vi "Update display.vi"(0 "This VI":refnum<vi>, 5 "Display":refnum<vi>, 9 "input":string, 11 "error in":errorcluster) -> (4 "Display out":string[][](array[string]), 6 "Location Cluster out":T1, 8 "Display array":string[][](array[string]), 10 "Display string":string, 15 "Error Out":errorcluster)   [LabVIEW 2018]
uses:
  location cluster.ctl
  CAEN globals.vi
panel:
  out "selected string":string
  out "Selection Position":cluster{i32, i32}
  out "Last cursor pos":cluster{i32, i32}
  out "Highlighted lines":i32[](array[numeric])
  out "Highlighted text":string[](array[string])
  out "sections":T2(array[cluster])
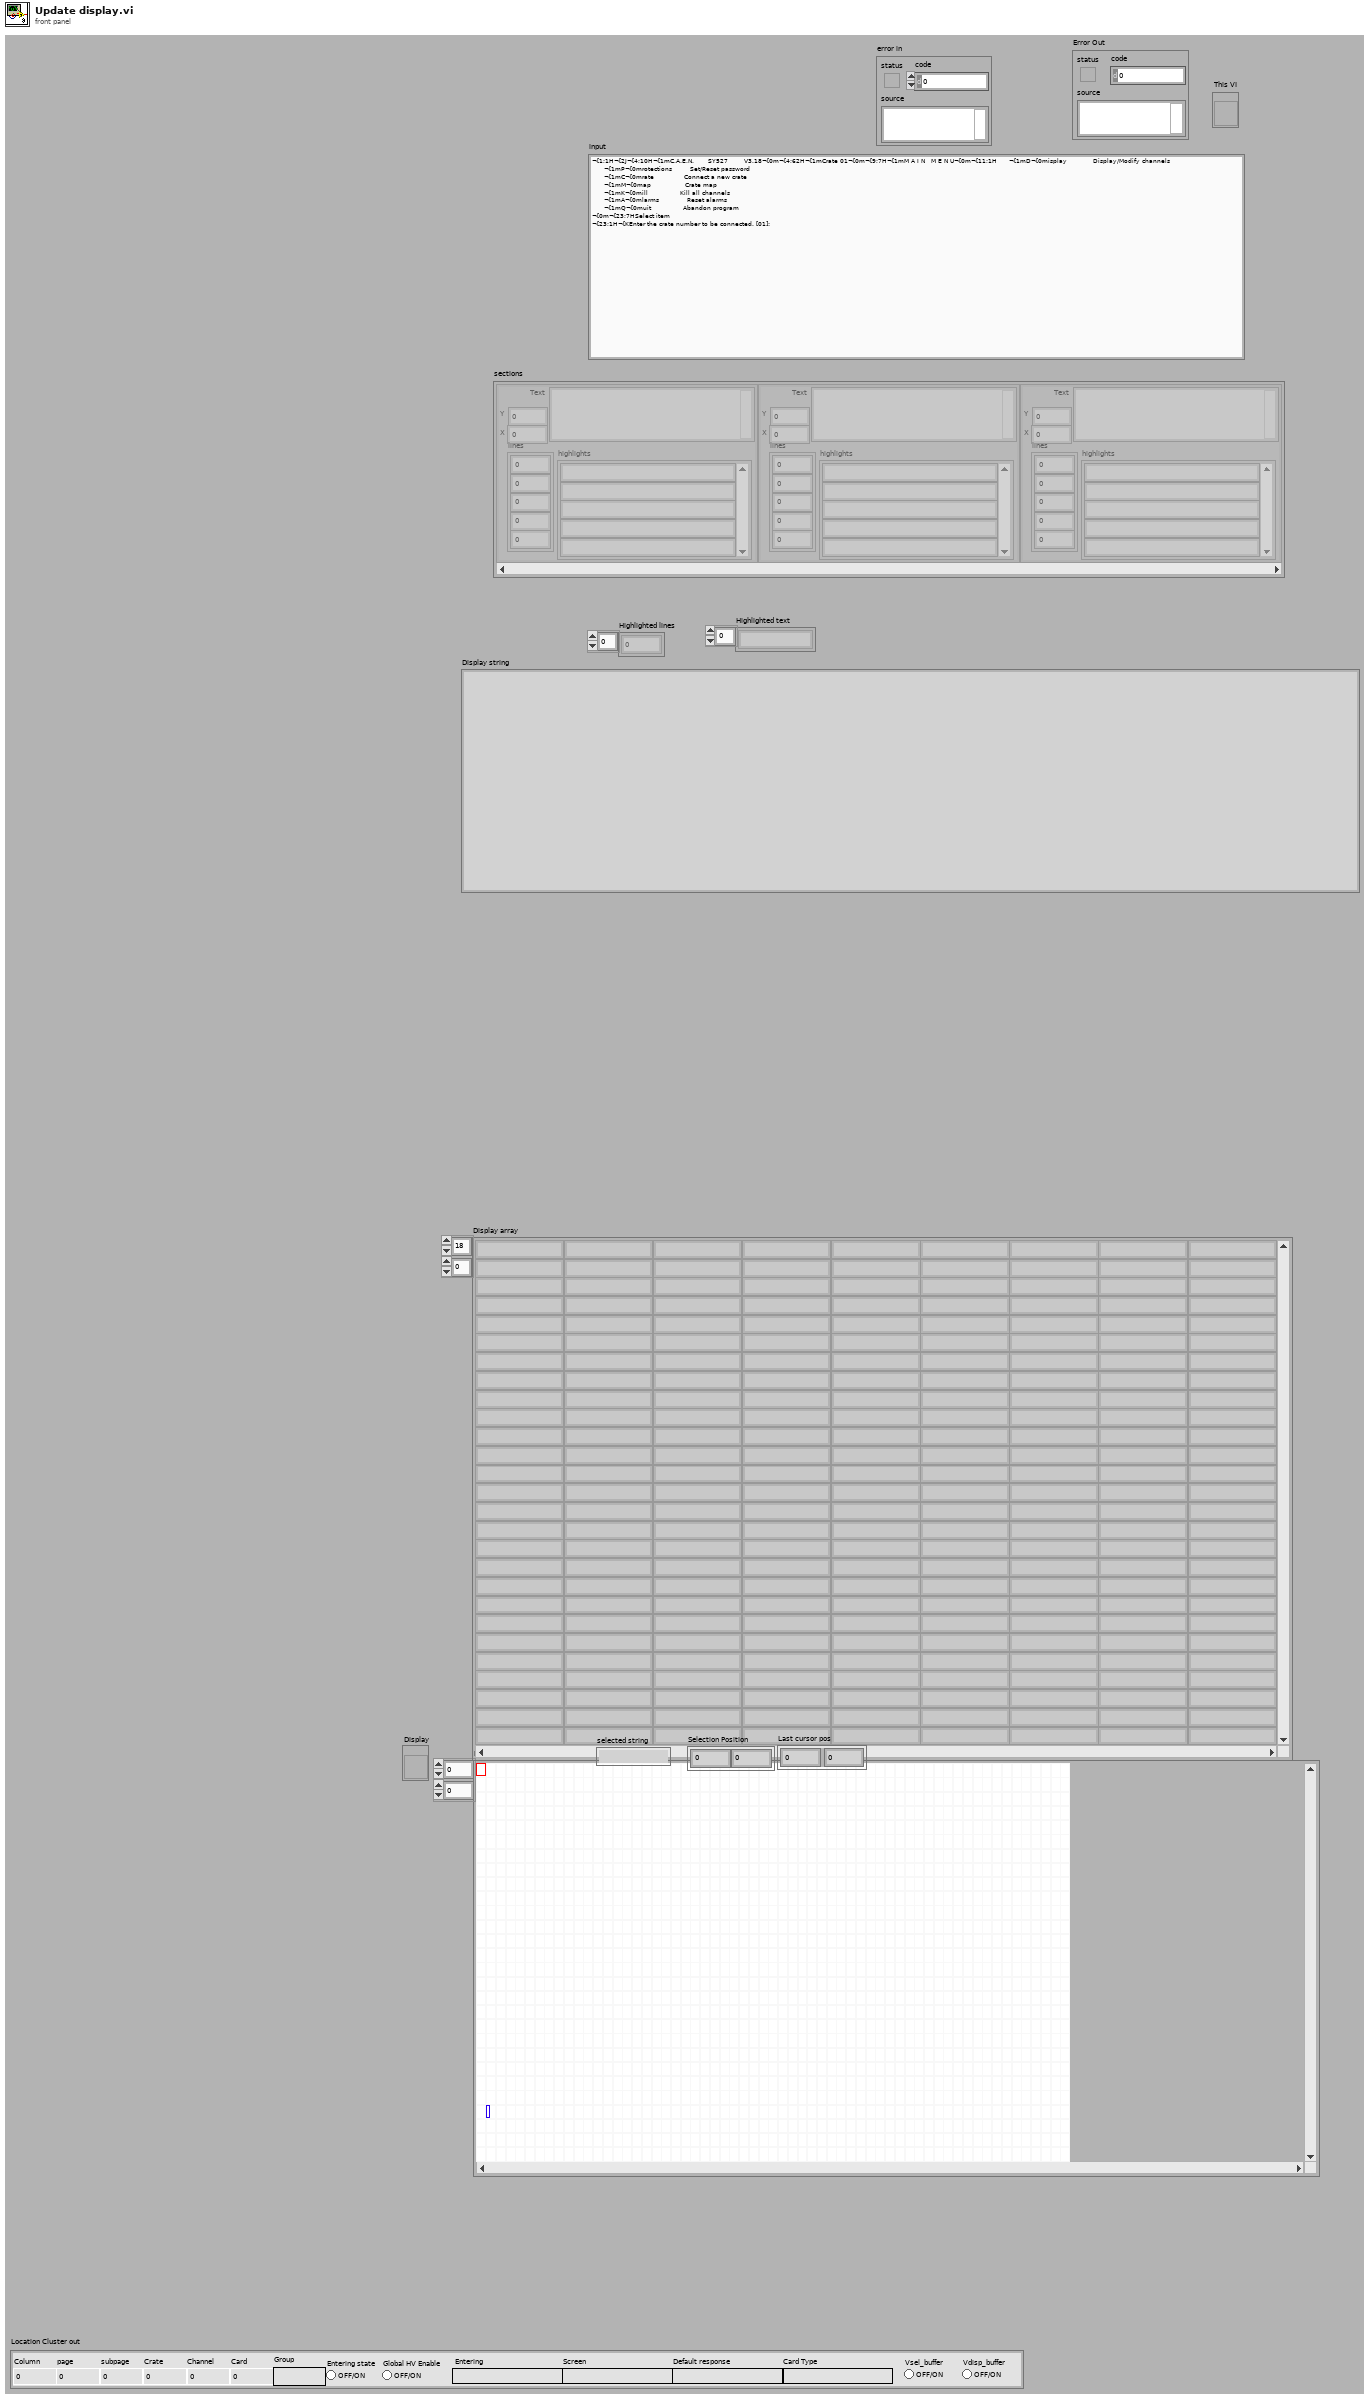
[diagram p1: front panel]
types:
  T1 = typedef "location cluster.ctl" = cluster{"Column":i32, "Card Type":string, "Channel":i32, "Card":i32, "Default response":string, "Entering":string, "Entering state":bool, "subpage":i32, "page":i32, "Crate":i32, "Screen":string, "Group":string, "Global HV Enable":bool, "Vsel_buffer":bool, "Vdisp_buffer":bool}
  T2 = cluster{"Y":i32, "X":i32, "Text":string, "highlights":string[], "lines":i32[]}[]
  T3 = cluster{"Y":i32, "X":i32, "stripped output":string, "highlighted strings":string[], "highlighted lines":i32[]}[]
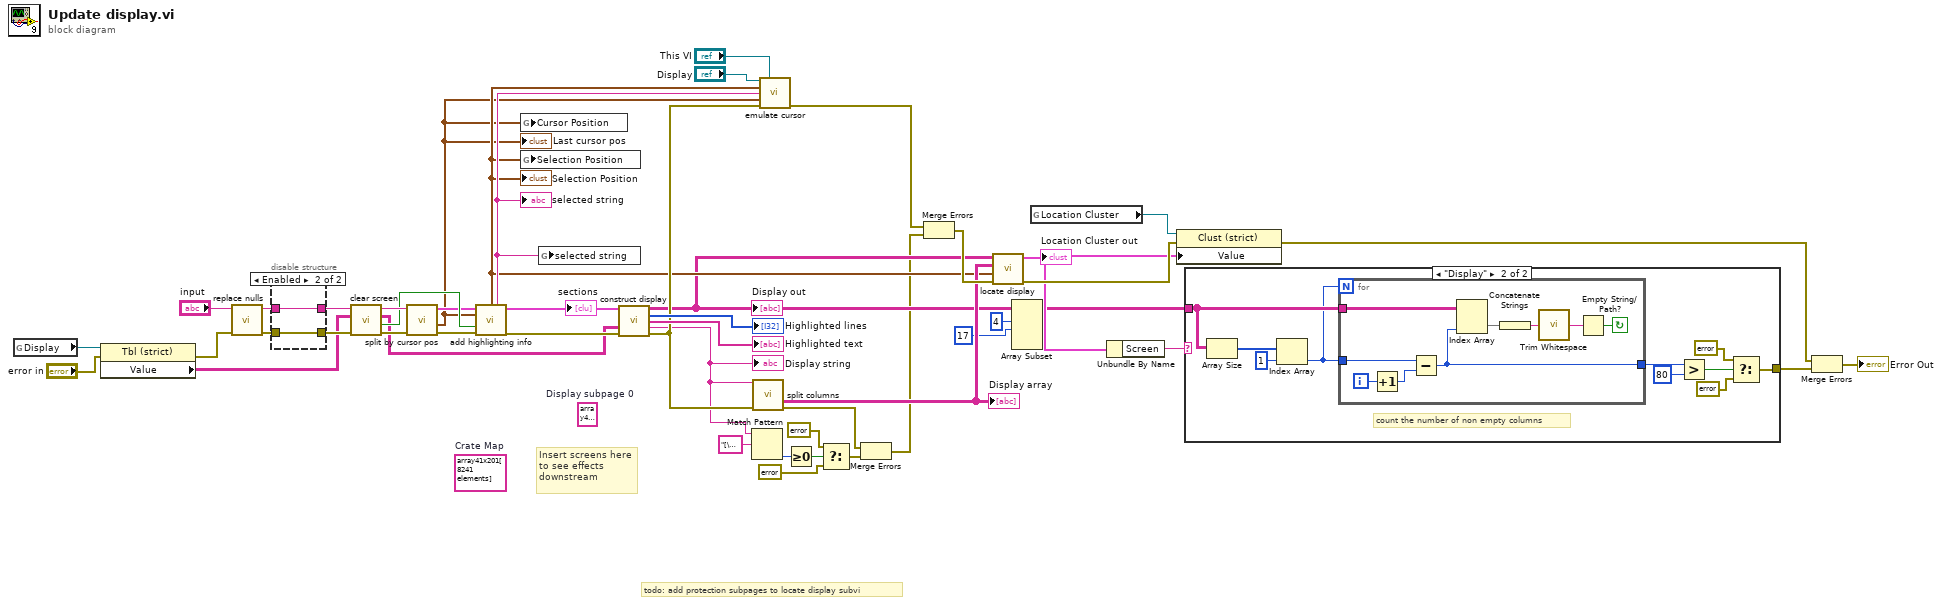
[diagram p0: block diagram]
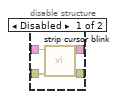
[diagram p2: hidden frame]
diagram:
  (unwired) string[][] array41x201[8241 elements]  # Crate Map
  (unwired) string[][] array41x201[8241 elements]  # Display subpage 0
  # "todo: add protection subpages to locate display subvi"
  # "Insert screens here\nto see effects\ndownstream"
  n1 = global read "CAEN globals.vi" "Display"() -> (w33:refnum<vi>)
  n2 = property class="Tbl (strict)"(reference=w33, error in="error in") -> (error out=w31:errorcluster, "Value"=w30:string[][])  [unwired: 1 out]
  n3 = call "replace nulls.vi"("error in (no error)"=w31, "read buffer"="input") -> ("error out"=w45:errorcluster, "result string"=w21:string)  [unwired: 8 in]
  n4 = disable-structure shown="Enabled" {
    disable-tunnel: w45 -> [w52 w53]
    disable-tunnel: [w51 w53] -> w44
    disable-tunnel: w21 -> [w50 w54]
    disable-tunnel: [w49 w54] -> w2
    frame Disabled {
      n5 = call "strip cursor blink.vi"("error in"=w52, "input"=w50) -> ("error out"=w51:errorcluster, "result string"=w49:string)  [unwired: 8 in]
    }
    frame Enabled {
    }
  }
  n6 = call "clear screen.vi"("error in"=w44, "Display in 2"=w30, "result string"=w2) -> ("error out"=w43:errorcluster, "Screen Cleared"=w39:bool, "Display in"=w34:string[][], "String"=w46:string)  [unwired: 1 in]
  n7 = call "split by cursor pos.vi"("error in"=w43, "input"=w46) -> ("error out"=w48:errorcluster, "Last cursor pos"=w1:cluster{i32, i32}, "data"=w22:cluster{"Y":i32, "X":i32, "Text":string}[])  [unwired: 6 in, 1 out]
  "Last cursor pos" <- w1
  n8 = call "add highlighting info.vi"("data"=w22, "Cursor Position"=w1, "Reset Selection"=w39, "error out"=w48) -> ("Selection Position"=w23:cluster{i32, i32}, "selected string"=w24:string, "Array"=w36:T3, "error IO"=w35:errorcluster)  [unwired: 6 in, 2 out]
  "sections" <- w36
  "Selection Position" <- w23
  "selected string" <- w24
  n9 = global write "CAEN globals.vi" "Cursor Position"(w1) -> ()
  n10 = global write "CAEN globals.vi" "Selection Position"(w23) -> ()
  n11 = global write "CAEN globals.vi" "selected string"(w24) -> ()
  n12 = call "construct display.vi"("input"=w36, "Display in"=w34, "error in"=w35) -> ("Display out"=w15:string[][], "Highlighted lines"=→"Highlighted lines":i32[], "Highlighted text"=→"Highlighted text":string[], "spreadsheet string"=w5:string, "error out"=w25:errorcluster)  [unwired: 6 in, 2 out]
  "Display string" <- w5
  "Display out" <- w15
  n13 = Match Pattern(string=w5, regular expression="[\u001b;]") -> (offset past match=w10:i32)  [unwired: 1 in, 3 out]
  n14 = call "split columns.vi"("Display string"=w5, "error in"=w25) -> ("Array"=w38:string[][], "error out"=w4:errorcluster)  [unwired: 9 in, 3 out]
  "Display array" <- w38
  n15 = call "emulate cursor.vi"("Display"="Display", "This VI"="This VI", "Selection"=w23, "Highlighted String"=w24, "Cursor"=w1, "error in"=w25) -> ("error out"=w26:errorcluster)  [unwired: 9 in]
  n16 = Greater Or Equal To 0?(x=w10) -> (x >= 0?=w9:bool)
  n17 = Select(t=errorcluster {"status"=TRUE, "code"=0, "source"="Corrupt characters present in read string!"}, s=w9, f=errorcluster {"status"=FALSE, "code"=0, "source"=""} ("t")) -> (s? t:f=w6:errorcluster)
  n18 = Merge Errors(w4, w6) -> (w3:errorcluster)
  n19 = Merge Errors(w26, w3) -> (w40:errorcluster)
  n20 = call "locate display.vi"("error in"=w40, "Selection Position"=w23, "Display array"=w38, "Display"=w15) -> ("error out"=w28:errorcluster, "Location Cluster out"=w17:T1)  [unwired: 6 in]
  "Location Cluster out" <- w17
  n21 = Array Subset(array=w15, index (row)=4 ("index"), length (row)=17 ("index")) -> (w14:string[][])  [unwired: 2 in]
  n22 = global read "CAEN globals.vi" "Location Cluster"() -> (w29:refnum<vi>)
  n23 = Unbundle By Name(w17) -> ("Screen"=w16:string)
  n24 = property class="Clust (strict)"(reference=w29, error in=w28, "Value"=w17) -> (error out=w19:errorcluster)  [unwired: 1 out]
  n25 = case shown="\"Display\"" w16 {
    tunnel: [_ w61] -> w20
    tunnel: w14 -> [_ w60]
    frame Default {
    }
    frame "Display" {
      # "count the number of non empty columns"
      n26 = Array Size(array=w60) -> (size(s)=w58:i32[])
      n27 = Index Array(array=w58, index=1) -> (element=w57:i32)
      n28 = for {
        N: w57 -> [_]
        tunnel: w60 -> [w73]
        tunnel: w57 -> [w72]
        tunnel: [w65] -> w56
        i -> [w71]
        stop <- w67 continue-if-true
        n29 = Increment(x=w71) -> (x+1=w66:i32)
        n30 = Subtract(x=w72, y=w66) -> (x-y=w65:i32)
        n31 = Index Array(array=w73, index (col)=w65) -> (element=w70:string[])  [unwired: 1 in]
        n32 = Concatenate Strings(w70) -> (w69:string)
        n33 = call <vilib>:"Trim Whitespace.vi"("string"=w69) -> ("trimmed string"=w68:string)  [unwired: 1 in]
        n34 = Empty String/Path?(string/path=w68) -> (empty?=w67:bool)
      }
      n35 = Greater?(x=w56, y=80) -> (0:w63:bool)
      n36 = Select(t=errorcluster {"status"=TRUE, "code"=0, "source"="Bad screen column count!"} ("error out"), s=w63, f=errorcluster {"status"=FALSE, "code"=0, "source"=""} ("error out")) -> (s? t:f=w61:errorcluster)
    }
  }
  n37 = Merge Errors(w19, w20) -> (→"Error Out":errorcluster)
